vi "thorlabs_write_serial.vi"(8 "error in (no error)":errorcluster, 10 "serial":string, 11 "thorlabs_kinesis in":refnum<class "thorlabs_kinesis.lvclass">) -> (0 "error out":errorcluster, 3 "thorlabs_kinesis out":refnum<class "thorlabs_kinesis.lvclass">)   [LabVIEW 2015, in "thorlabs_kinesis.lvclass"]
uses:
  thorlabs_kinesis.lvclass
  thorlabs_kinesis.lvclass/thorlabs_kinesis.ctl
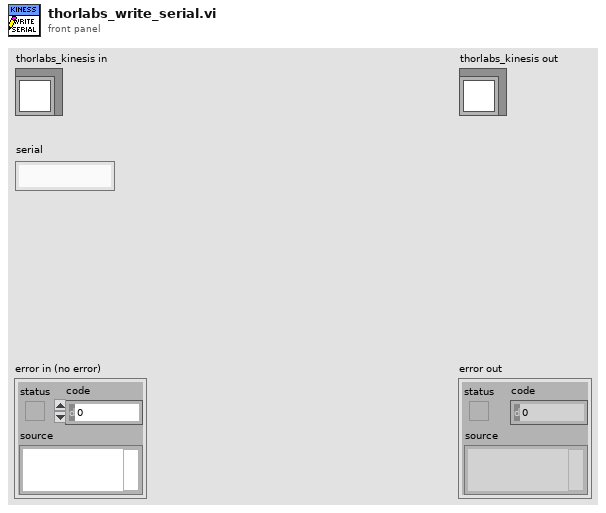
[diagram p1: front panel]
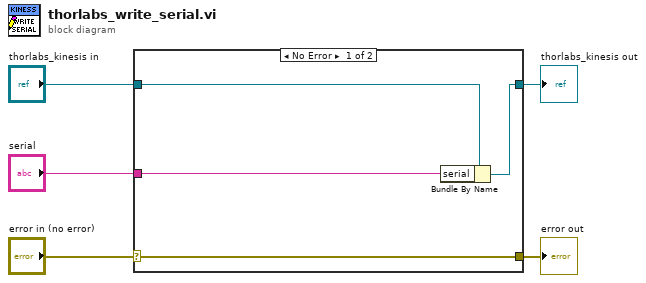
[diagram p0: block diagram]
diagram:
  n1 = case shown="No Error" "error in (no error)" {
    selector: "error in (no error)" -> [w9 w10]
    tunnel: [w9 w10] -> w4
    tunnel: [w7 w11] -> w2
    tunnel: "thorlabs_kinesis in" -> [w8 w11]
    tunnel: "serial" -> [w6 _]
    frame No Error {
      n2 = Bundle By Name(cluster=w8, "serial"=w6) -> (w7:refnum<class "thorlabs_kinesis.lvclass">)
    }
    frame Error {
    }
  }
  "error out" <- w4
  "thorlabs_kinesis out" <- w2
